vi "Draw.vi"(8 "error in (no error)":errorcluster, 10 "2D Picture in":picture, 11 "Shape in":refnum<class "Shape.lvclass">) -> (0 "error out":errorcluster, 2 "2D Picture out":picture, 3 "Shape out":refnum<class "Shape.lvclass">)   [LabVIEW 2021, in "Picture2D.lvlib" / "Shape.lvclass"]
uses:
  Shape.lvclass
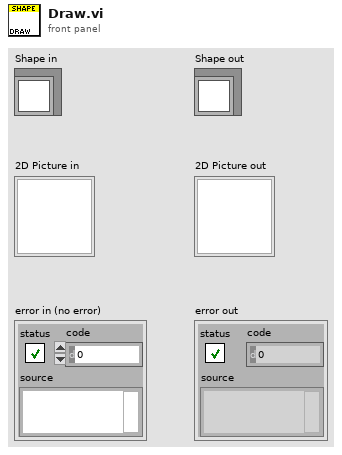
[diagram p1: front panel]
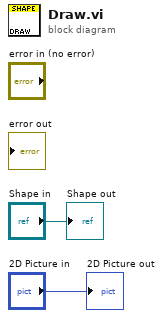
[diagram p0: block diagram]
diagram:
  "Shape out" <- "Shape in"
  "2D Picture out" <- "2D Picture in"
